vi "sub_main_data-process.vi"(8 "error in":errorcluster) -> (0 "error out":errorcluster)   [LabVIEW 2019]
uses:
  Ctrl/pid-in-params.ctl
  Ctrl/points.ctl
panel:
  out "dt s":dbl
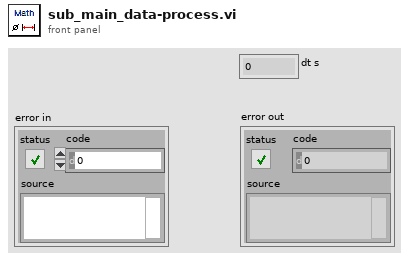
[diagram p1: front panel]
types:
  T1 = typedef "pid-in-params.ctl" = enum16{"read", "write"}
  T2 = typedef "points.ctl" = enum16{"read", "lookahead circle in", "lookahead in", "looktail in", "center in"}
  T3 = cluster{"deg_agv-lookahead":dbl, "deg_waypoint":dbl, "deg_gap":dbl, "deg_target":dbl, "pid output":dbl, "distance-gap_out":dbl}
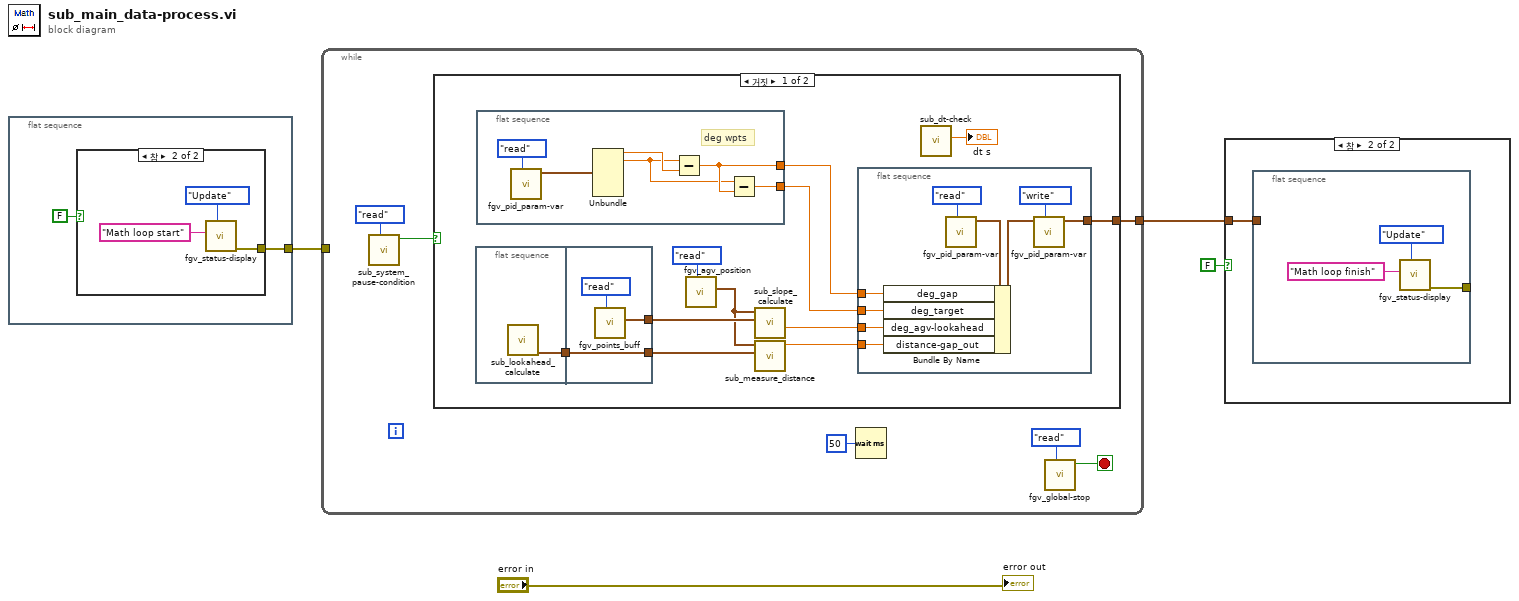
[diagram p0: block diagram]
diagram:
  n1 = flat-sequence {
    tunnel: [w6] -> w3
    frame #0 {
      n2 = case shown="참" FALSE {
        tunnel: [_ w7] -> w6
        frame False {
        }
        frame True {
          n3 = call "fgv_status-display.vi"("Mode"=enum16{"Initial", "Update", "Clear"}."Update", "title"="Math loop start" ("String in 1")) -> ("error out"=w7:errorcluster)  [unwired: 9 in]
        }
      }
    }
  }
  n4 = while {
    tunnel: w3 -> [_]
    tunnel: [w14] -> w2
    stop <- w12 stop-if-true
    n5 = call "sub_system_pause-condition.vi"("cmd"=enum16{"pause", "go", "read"}."read") -> ("pause"=w10:bool)  [unwired: 10 in]
    n6 = case shown="거짓" w10 {
      tunnel: [w17 _] -> w14
      frame False {
        n7 = flat-sequence {
          tunnel: [w42] -> w26
          tunnel: [w44] -> w24
          tunnel: [w43] -> w23
          tunnel: w26 -> [w43]
          frame #0 {
            n8 = call "sub_lookahead_calculate.vi"() -> ("center point"=w42:cluster{"x":dbl, "y":dbl})  [unwired: 7 in, 4 out]
          }
          frame #1 {
            n9 = call "fgv_points_buff.vi"("cmd"=points."read") -> ("lookahead out"=w44:cluster{"x":dbl, "y":dbl})  [unwired: 7 in, 3 out]
          }
        }
        n10 = flat-sequence {
          tunnel: [w38] -> w22
          tunnel: [w37] -> w21
          frame #0 {
            # "deg wpts"
            n11 = call "fgv_pid_param-var.vi"("cmd"=pid-in-params."read") -> ("pid-var_output"=w40:T3)  [unwired: 10 in]
            n12 = Unbundle(w40) -> ("deg_agv-lookahead"=w39:dbl, "deg_waypoint"=w36:dbl)  [unwired: 4 out]
            n13 = Subtract(x=w36, y=w39) -> (x-y=w38:dbl)
            n14 = Subtract(x=w36, y=w38) -> (x-y=w37:dbl)
          }
        }
        n15 = call "fgv_agv_position.vi"("cmd"=enum16{"write", "read"}."read") -> ("utm out"=w16:cluster{dbl, dbl})  [unwired: 8 in, 2 out]
        n16 = call "sub_slope_calculate.vi"("point n+1"=w24, "point n"=w16) -> ("deg_gps-base"=w19:dbl)  [unwired: 7 in, 2 out]
        n17 = call "sub_measure_distance.vi"("pt 2"=w23, "pt 1"=w16) -> ("distance"=w20:dbl)  [unwired: 9 in]
        n18 = flat-sequence {
          tunnel: w22 -> [w32]
          tunnel: w21 -> [w31]
          tunnel: w20 -> [w30]
          tunnel: w19 -> [w28]
          tunnel: [w27] -> w17
          frame #0 {
            n19 = call "fgv_pid_param-var.vi"("cmd"=pid-in-params."read") -> ("pid-var_output"=w33:T3)  [unwired: 10 in]
            n20 = Bundle By Name(cluster=w33, "deg_gap"=w32, "deg_target"=w31, "deg_agv-lookahead"=w28, "distance-gap_out"=w30) -> (w29:T3)
            n21 = call "fgv_pid_param-var.vi"("cmd"=pid-in-params."write", "pid-vars_in"=w29) -> ("pid-var_output"=w27:T3)  [unwired: 9 in]
          }
        }
        n22 = call "sub_dt-check.vi"() -> ("dt s"=→"dt s":dbl)  [unwired: 10 in, 1 out]
      }
      frame True {
      }
    }
    n23 = Wait (ms)(milliseconds to wait=u32 50) -> ()  [unwired: 1 out]
    n24 = call "fgv_global-stop.vi"("cmd"=enum16{"init", "stop", "read"}."read") -> ("val_out"=w12:bool)  [unwired: 10 in]
  }
  n25 = case shown="참" FALSE {
    tunnel: w2 -> [_ w46]
    frame False {
    }
    frame True {
      n26 = flat-sequence {
        tunnel: [w47] -> _
        tunnel: w46 -> [_]
        frame #0 {
          n27 = call "fgv_status-display.vi"("Mode"=enum16{"Initial", "Update", "Clear"}."Update", "title"="Math loop finish" ("String in 1")) -> ("error out"=w47:errorcluster)  [unwired: 9 in]
        }
      }
    }
  }
  "error out" <- "error in"
